vi "PH_PILS.Action _Experiment.vi"(0 "i ref in":refnum<vi>, 5 "error IO":errorcluster) -> (14 "i ref out":refnum<vi>, 19 "error out":errorcluster)   [LabVIEW 2014, in "PH_PILS.lvlib"]
doc: "This Vi calculates the experimental mode."
uses:
  PH_PILS.lvlib
  PH_Common/PH_Common.lvlib
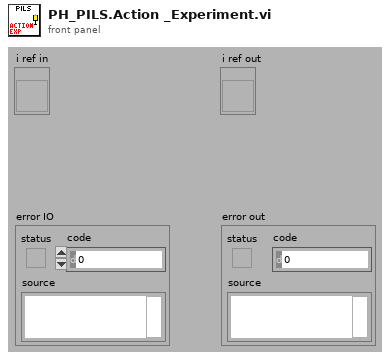
[diagram p1: front panel]
types:
  T1 = typedef "PH_PILS.lvlib/PH_PILS.i attribute.ctl" = cluster{"Boolean":cluster{"GUI Ref":refnum<vi>, "Status":i32}[], "GUI Refs Exp. Shutters":cluster{"1":refnum<vi>, "2":refnum<vi>, "3":refnum<vi>, "4":refnum<vi>}, "Tristate2Run GUI Refs":refnum<vi>[], "EO-Likes":cluster{"GUI Ref":refnum<vi>, "Status":i32}[], "Operation Mode":cluster{"Operation Mode":T2, "GUI":cluster{"Ref State":refnum<vi>, "Ref":refnum<vi>}, "Servicemode":cluster{"Tagname":string, "Status":i32}, "Labormode":cluster{"Tagname":string, "Status":i32}, "Searchmode":cluster{"Tagname":string, "Status":i32}, "Shotmode":cluster{"Tagname":string, "Status":i32}}, "Submode":cluster{"Submode":T3, "GUI":cluster{"Ref State":refnum<vi>, "Ref":refnum<vi>}, "Submode":cluster{"Tagname":string, "Status":i32}}, "Experiment":cluster{"Experiment":enum16{"unknown", "intern", "4 (Z6)", "3", "2", "1"}, "GUI":cluster{"Ref State":refnum<vi>, "Ref":refnum<vi>}, "intern":cluster{"Tagname":string, "Status":i32}, "Exp 4":cluster{"Tagname":string, "Status":i32}, "Exp 3":cluster{"Tagname":string, "Status":i32}, "Exp 2":cluster{"Tagname":string, "Status":i32}, "Exp 1":cluster{"Tagname":string, "Status":i32}}, "TristateNormal":cluster{"GUI Ref":refnum<vi>, "Status":i32}[], "Door Tags":cluster{"GUI Ref":refnum<vi>, "Status":i32}[], "GUIlessTags":cluster{"Name":string, "Status":i32}[], "Beamline GUI Refs":refnum<vi>[], "Special Boolean":cluster{"GUI Ref":refnum<vi>, "Status":i32}[], "Laserpower":cluster{"GUI Ref":refnum<vi>, "Status":i32}[], "Shutter":cluster{"GUI Ref":refnum<vi>, "Status":i32}[], "Tristate EO Like":cluster{"GUI Ref":refnum<vi>, "Status":i32}[], "PP":cluster{"GUI Ref":refnum<vi>, "Status":i32, "Head Ref":refnum<vi>, "Slider Ref":refnum<vi>}[], "Switch Knobs":cluster{"GUI Ref":refnum<vi>, "Status":i32}[], "Latch Knob GUI Refs":refnum<vi>[], "FailureCounter":i32, "Enabled Status":cluster{"Laser":i32, "PreAmp":i32, "MainAmp":i32}, "Mercury":refnum<vi>, "Instance Rods":string, "Logfile":path, "Beckhoff-Instance Internal":string, "Beckhoff-Instance External":string, "Enabling Rights":cluster{"Name":string, "Password":string, "PA?":bool, "MA?":bool, "Exp?":bool}[]}
  T2 = typedef "PH_PILS.lvlib/PH_PILS.Operation Mode.ctl" = enum16{"unknown", "Service", "Labor", "Search", "Shot"}
  T3 = typedef "PH_PILS.lvlib/PH_PILS.Submode.ctl" = enum16{"unknown", "HV-Normal", "HV-Test"}
  T4 = enum16{"unknown", "intern", "4 (Z6)", "3", "2", "1"}
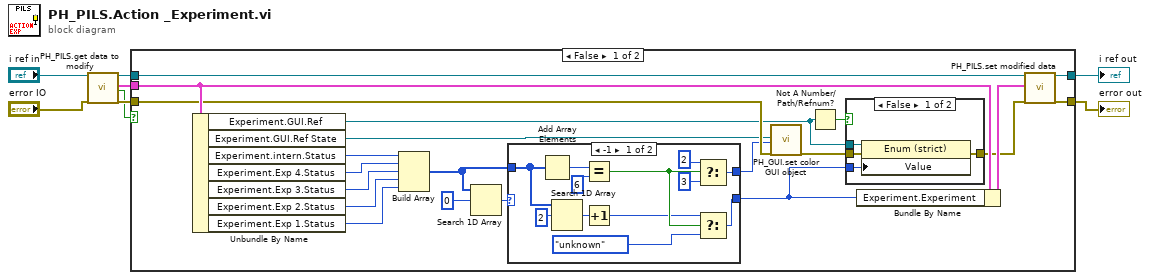
[diagram p0: block diagram]
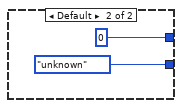
[diagram p2: hidden frame]
diagram:
  n1 = call "PH_PILS.get data to modify.vi"("i ref in"="i ref in", "error in (no error)"="error IO") -> ("i ref out"=w7:refnum<vi>, "i attribute"=w5:T1, "timed out"=w6:bool, "error out"=w8:errorcluster)  [unwired: 14 in]
  n2 = case shown="False" w6 {
    tunnel: [w29 w49] -> w3
    tunnel: w8 -> [w20 w49]
    tunnel: [w28 w50] -> w4
    tunnel: w7 -> [w27 w50]
    tunnel: w5 -> [w22 _]
    frame False {
      n3 = Unbundle By Name(w22) -> ("Experiment.GUI.Ref"=w15:refnum<vi>, "Experiment.GUI.Ref State"=w16:refnum<vi>, "Experiment.intern.Status"=w26:i32, "Experiment.Exp 4.Status"=w25:i32, "Experiment.Exp 3.Status"=w24:i32, "Experiment.Exp 2.Status"=w23:i32, "Experiment.Exp 1.Status"=w9:i32)
      n4 = Build Array(w26, w25, w24, w23, w9) -> (w10:i32[])
      n5 = Search 1D Array(1D array=w10, element=0) -> (index of element=w13:i32)  [unwired: 1 in]
      n6 = case shown="-1" w13 {
        tunnel: [w35 T4."unknown" ("Experiment.Experiment")] -> w12
        tunnel: [w38 0 ("State")] -> w11
        tunnel: w10 -> [w34 _]
        frame -1 {
          n7 = Add Array Elements(numeric array=w34) -> (sum=w41:i32)
          n8 = Search 1D Array(1D array=w34, element=2) -> (index of element=w33:i32)  [unwired: 1 in]
          n9 = Equal?(x=w41, y=6) -> (x = y?=w36:bool)
          n10 = Increment(x=w33) -> (x+1=w31:i32)
          n11 = Select(t=2 ("State"), s=w36, f=3) -> (s? t:f=w38:i32)
          n12 = Select(t=w31, s=w36, f=T4."unknown" ("Experiment.Experiment")) -> (s? t:f=w35:i32)
        }
        frame Default {
        }
      }
      n13 = call "PH_GUI.set color GUI object.vi"("GUI object Ref"=w16, "State"=w11, "error in (no error)"=w20) -> ("error out"=w17:errorcluster)  [unwired: 16 in]
      n14 = Not A Number/Path/Refnum?(number/path/refnum=w15) -> (NaN/Path/Refnum?=w18:bool)
      n15 = case shown="False" w18 {
        tunnel: w17 -> [w47 w48]
        tunnel: [w46 w48] -> w19
        tunnel: w15 -> [w45 _]
        tunnel: w12 -> [w44 _]
        frame False {
          n16 = property class="Enum (strict)"(reference=w45, error in=w47, "Value"=w44) -> (error out=w46:errorcluster)  [unwired: 1 out]
        }
        frame True {
        }
      }
      n17 = Bundle By Name(cluster=w22, "Experiment.Experiment"=w12) -> (w21:T1)
      n18 = call "PH_PILS.set modified data.vi"("i ref in"=w27, "i attribute"=w21, "error in (no error)"=w19) -> ("i ref out"=w28:refnum<vi>, "error out"=w29:errorcluster)  [unwired: 15 in]
    }
    frame True {
    }
  }
  "error out" <- w3
  "i ref out" <- w4
